vi "Set Channel Values Block Data Ref.vi"(8 "error in":errorcluster, 9 "Values Array in":dbl[](array[numeric]), 10 "Block Data Ref":T1[](array[typedef]) {"Data Reference" format="%.0x"}, 11 "VS Engine Interface in":refnum<class "VS Engine Interface.lvclass">) -> (0 "error out":errorcluster, 1 "Values Array out":dbl[](array[numeric]), 2 "Block Data Ref dup":T1[](array[typedef]) {"Data Reference" format="%.0x"}, 3 "VS Engine Interface out":refnum<class "VS Engine Interface.lvclass">)   [LabVIEW 2024, in "VS Engine Abstraction.lvlib" / "VS Engine Interface.lvclass"]
uses:
  VS Engine Interface.lvclass
  <vilib>/NI VeriStand/Custom Device API/Data Reference.ctl
  <vilib>/NI VeriStand/Custom Device API/Custom Device API.lvlib
  <vilib>/NI VeriStand/Custom Device API/Block Data Reference.ctl
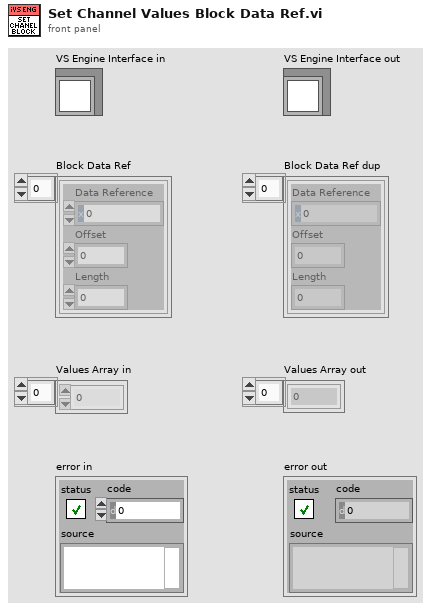
[diagram p1: front panel]
types:
  T1 = typedef "Custom Device API.lvlib/Block Data Reference.ctl" = cluster{"Data Reference":T2, "Offset":u64, "Length":u64}
  T2 = typedef "Custom Device API.lvlib/Data Reference.ctl" = i32
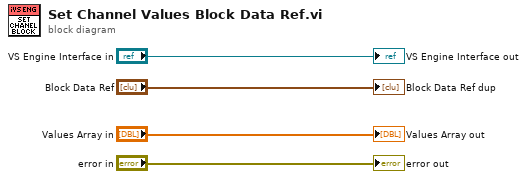
[diagram p0: block diagram]
diagram:
  "error out" <- "error in"
  "VS Engine Interface out" <- "VS Engine Interface in"
  "Values Array out" <- "Values Array in"
  "Block Data Ref dup" <- "Block Data Ref"
